vi "Encoder Test.vi"() -> ()   [LabVIEW 2011]
uses:
  <vilib>/Rock Robotics/SystemInterfaces/DIO/FPGA_DIOChannel.ctl
  <vilib>/Rock Robotics/SystemInterfaces/DIO/FPGA_DIOPWMChannel.ctl
  <vilib>/Rock Robotics/WPI/Joystick/WPI_JoystickDeviceEnum.ctl
  <vilib>/Rock Robotics/WPI/Encoder/WPI_EncoderType.ctl
  <vilib>/Rock Robotics/SystemInterfaces/Typedef/FPGA_TypedefDigitalModule.ctl
  <vilib>/Rock Robotics/SystemInterfaces/Typedef/FPGA_TypedefAnalogModule.ctl
  <vilib>/Rock Robotics/SystemInterfaces/AI/FPGA_AIChannel.ctl
  <vilib>/Rock Robotics/WPI/Counter/WPI_CounterDigitalInputToDigitalSource.vi
  <vilib>/Rock Robotics/WPI/MotorControl/WPI_MotorControlOpen Jaguar.vi
  <vilib>/Rock Robotics/WPI/Counter/WPI_CounterOpen UpDown Mode.vi
panel:
  out "period":dbl
  out "Numeric":dbl
  out "Average":dbl
  out "Voltage":dbl(knob) scale=30.0..80.0
  out "RPM 2":dbl(knob) scale=0.0..6000.0
  in  "Knob":dbl(knob) scale=0.0..1.0
  out "Gauge 2":dbl(knob) scale=-100.0..100.0
  in  "stop":bool
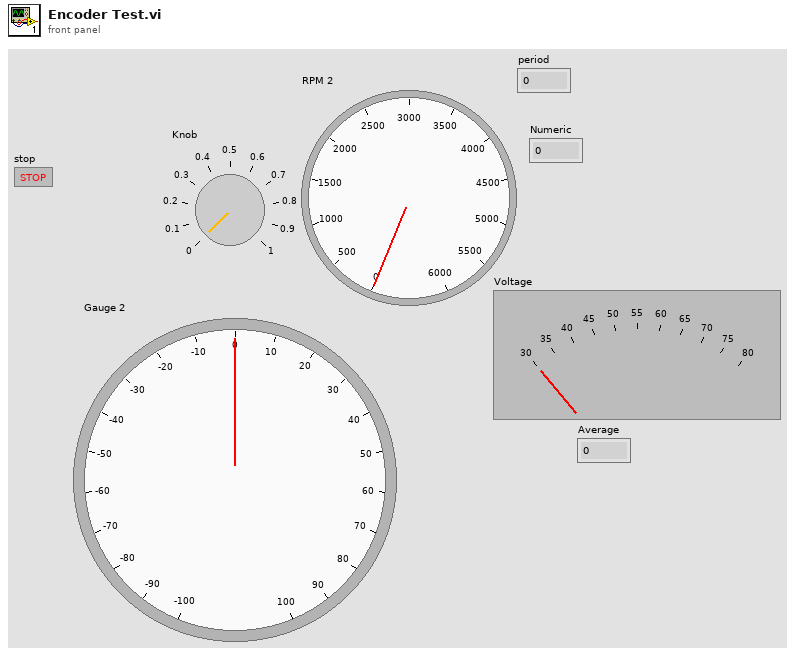
[diagram p1: front panel]
types:
  T1 = typedef "FPGA_AIChannel.ctl" = enum8{"AI 1", "AI 2", "AI 3", "AI 4", "AI 5", "AI 6", "AI 7", "AI 8", "Invalid"}
  T2 = typedef "FPGA_TypedefAnalogModule.ctl" = enum16{"Analog Module 1", "Analog Module 2"}
  T3 = typedef "FPGA_DIOChannel.ctl" = enum8{"DIO 1", "DIO 2", "DIO 3", "DIO 4", "DIO 5", "DIO 6", "DIO 7", "DIO 8", "DIO 9", "DIO 10", "DIO 11", "DIO 12", "DIO 13", "DIO 14", "Invalid"}
  T4 = typedef "FPGA_TypedefDigitalModule.ctl" = enum16{"Digital Module 1", "Digital Module 2"}
  T5 = typedef "WPI_EncoderType.ctl" = enum16{"1x", "2x", "4x"}
  T6 = typedef "FPGA_DIOPWMChannel.ctl" = enum8{"PWM 1", "PWM 2", "PWM 3", "PWM 4", "PWM 5", "PWM 6", "PWM 7", "PWM 8", "PWM 9", "PWM 10", "Invalid"}
  T7 = typedef "WPI_JoystickDeviceEnum.ctl" = enum16{"USB 1", "USB 2", "USB 3", "USB 4", "Kinect 1", "Kinect 2"}
  T8 = typedef "WPI_DigitalInputDevRef.ctl" = cluster{"DevStatus":errorcluster, "DIO Channel":T3, "Digital Module":T4}
  T9 = typedef "FPGA_CounterEncoderSourceConvertionLVSourceType.ctl" = cluster{"DevStatus":errorcluster, "AnalogTriggerMode?":bool, "DigitalMode":cluster{"Digital Module":T4, "DIO Channel":T10}, "AnalogTriggerMode":cluster{"AnalogTriggerIndex":T11, "OutputType":T12}}
  T10 = typedef "FPGA_DIODigitalSourceChannel.ctl" = enum8{"DIO 1", "DIO 2", "DIO 3", "DIO 4", "DIO 5", "DIO 6", "DIO 7", "DIO 8", "DIO 9", "DIO 10", "DIO 11", "DIO 12", "DIO 13", "DIO 14", "Disabled"}
  T11 = typedef "FPGA_AnalogTriggerIndex.ctl" = enum8{"Trig 0", "Trig 1", "Trig 2", "Trig 3", "Trig 4", "Trig 5", "Trig 6", "Trig 7", "Invalid"}
  T12 = typedef "FPGA_AnalogTriggerOutType.ctl" = enum16{"InWindow", "TriggerState", "Rising", "Falling"}
  T13 = typedef "WPI_EncoderDevRef.ctl" = cluster{"DevStatus":errorcluster, "EncoderIndex":T14, "CounterIndex":T15, "DistancePerCount":dbl, "Decoding Type":T5}
  T14 = typedef "FPGA_EncoderIdx.ctl" = enum8{"Enc 0", "Enc 1", "Enc 2", "Enc 3", "Invalid"}
  T15 = typedef "FPGA_CounterCtrSystemIndex.ctl" = enum8{"Ctr 0", "Ctr 1", "Ctr 2", "Ctr 3", "Ctr 4", "Ctr 5", "Ctr 6", "Ctr 7", "Invalid"}
  T16 = typedef "WPI_CounterDevRef.ctl" = cluster{"DevStatus":errorcluster, "CntIndex":T15}
  T17 = typedef "WPI_MotorControlDeviceRef.ctl" = cluster{"DeviceStatus":errorcluster, "Type":enum16{"PWM", "CAN"}, "PWM":cluster{"Digital Module":T4, "PWM Channel":T6, "DeadBand":T18}, "CAN":cluster{"Device Number":u8, "Control Mode":T19, "Semaphore":T20, "Max Vout":dbl}, "Invert":bool, "TransformRef":T21, "InvTransformRef":T21}
  T18 = typedef "WPI_PWMDeadband.ctl" = cluster{"Name":string, "maxPositivePwm":i32, "minPositivePwm":i32, "centerPwm":i32, "maxNegativePwm":i32, "minNegativePwm":i32, "angularRange":u16}
  T19 = typedef "WPI_CANJaguar_ControlMode.ctl" = enum8{"Percent VBus", "Current", "Speed", "Position", "Voltage"}
  T20 = typedef "Semaphore RefNum" = refnum<k1>
  T21 = typedef "WPI_PWMTransform_ConPane.ctl" = refnum<vi>
  T22 = typedef "WPI_AnalogChannelDevRef.ctl" = cluster{"DevStatus":errorcluster, "Analog Module":T2, "Analog Channel":T1}
  T23 = typedef "WPI_JoystickDevRef.ctl" = cluster{"Device":T7}
  T24 = typedef "WPI_JoystickButtonState.ctl" = cluster{"Button 1":bool, "Button 2":bool, "Button 3":bool, "Button 4":bool, "Button 5":bool, "Button 6":bool, "Button 7":bool, "Button 8":bool, "Button 9":bool, "Button 10":bool, "Button 11":bool, "Button 12":bool}
  T25 = cluster{"axis 1 (x)":dbl, "axis 2 (y)":dbl, "axis 3 (throttle)":dbl, "axis 4":dbl, "axis 5":dbl, "axis 6":dbl}
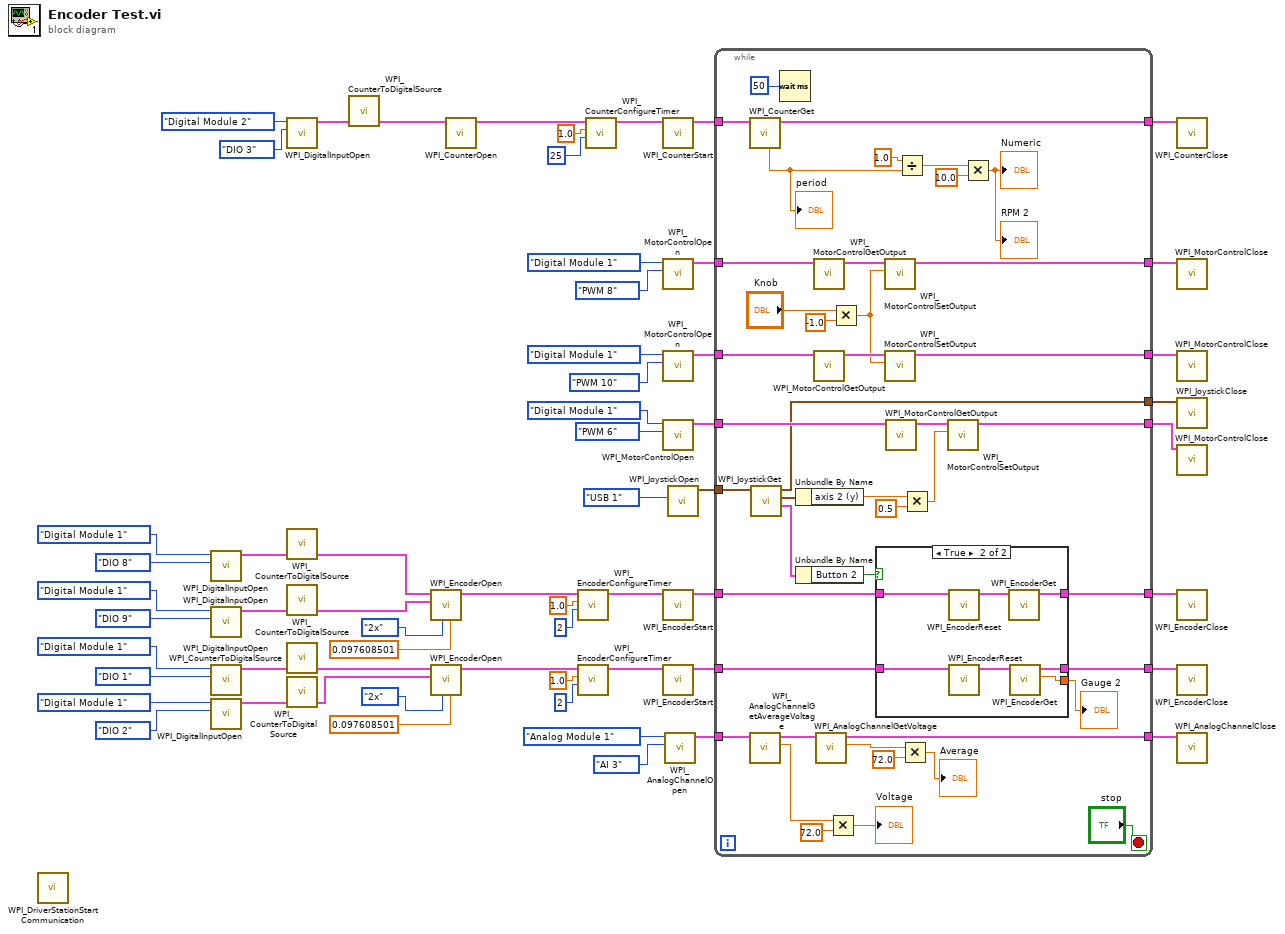
[diagram p0: block diagram]
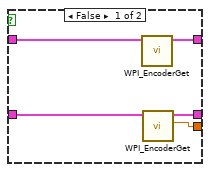
[diagram p2: hidden frame]
diagram:
  n1 = call <vilib>:"WPI_DriverStationStart Communication.vi"() -> ()  [unwired: 12 in]
  n2 = call <vilib>:"WPI_DigitalInputOpen.vi"("DIO Channel"=FPGA_DIOChannel."DIO 8", "Digital Module (Module 1)"=FPGA_TypedefDigitalModule."Digital Module 1") -> ("DigitalInputDevRef"=w58:T8)  [unwired: 8 in, 1 out]
  n3 = call <vilib>:"WPI_DigitalInputOpen.vi"("DIO Channel"=FPGA_DIOChannel."DIO 9", "Digital Module (Module 1)"=FPGA_TypedefDigitalModule."Digital Module 1") -> ("DigitalInputDevRef"=w61:T8)  [unwired: 8 in, 1 out]
  n4 = call <vilib>:"WPI_DigitalInputOpen.vi"("DIO Channel"=FPGA_DIOChannel."DIO 1", "Digital Module (Module 1)"=FPGA_TypedefDigitalModule."Digital Module 1") -> ("DigitalInputDevRef"=w22:T8)  [unwired: 8 in, 1 out]
  n5 = call <vilib>:"WPI_DigitalInputOpen.vi"("DIO Channel"=FPGA_DIOChannel."DIO 2", "Digital Module (Module 1)"=FPGA_TypedefDigitalModule."Digital Module 1") -> ("DigitalInputDevRef"=w19:T8)  [unwired: 8 in, 1 out]
  n6 = call <vilib>:"WPI_DigitalInputOpen.vi"("DIO Channel"=FPGA_DIOChannel."DIO 3", "Digital Module (Module 1)"=FPGA_TypedefDigitalModule."Digital Module 2") -> ("DigitalInputDevRef"=w11:T8)  [unwired: 8 in, 1 out]
  n7 = call-poly <vilib>:"WPI_CounterToDigitalSource.vi"("DigitalInputDevRef"=w58) -> ("Digital Source"=w59:T9)  [unwired: 6 in]
  n8 = call-poly <vilib>:"WPI_CounterToDigitalSource.vi"("DigitalInputDevRef"=w61) -> ("Digital Source"=w60:T9)  [unwired: 6 in]
  n9 = call-poly <vilib>:"WPI_CounterToDigitalSource.vi"("DigitalInputDevRef"=w22) -> ("Digital Source"=w21:T9)  [unwired: 6 in]
  n10 = call-poly <vilib>:"WPI_CounterToDigitalSource.vi"("DigitalInputDevRef"=w19) -> ("Digital Source"=w20:T9)  [unwired: 6 in]
  n11 = call-poly <vilib>:"WPI_CounterToDigitalSource.vi"("DigitalInputDevRef"=w11) -> ("Digital Source"=w12:T9)  [unwired: 6 in]
  n12 = call <vilib>:"WPI_EncoderOpen.vi"("DistancePerCount"=0.097608501, "Decoding Type"=WPI_EncoderType."2x", "BSource"=w60, "ASource"=w59) -> ("EncoderDevRef"=w53:T13)  [unwired: 6 in, 1 out]
  n13 = call <vilib>:"WPI_EncoderOpen.vi"("DistancePerCount"=0.097608501, "Decoding Type"=WPI_EncoderType."2x", "BSource"=w20, "ASource"=w21) -> ("EncoderDevRef"=w27:T13)  [unwired: 6 in, 1 out]
  n14 = call-poly <vilib>:"WPI_CounterOpen.vi"("Up Source"=w12) -> ("CounterDevRef"=w16:T16)  [unwired: 9 in, 1 out]
  n15 = call <vilib>:"WPI_EncoderConfigureTimer.vi"("Number Samples to Average"=u8 2, "Minimum Rate"=1.0, "EncoderDevRef"=w53) -> ("EncoderDevRef"=w52:T13)  [unwired: 7 in, 1 out]
  n16 = call <vilib>:"WPI_EncoderConfigureTimer.vi"("Number Samples to Average"=u8 2, "Minimum Rate"=1.0, "EncoderDevRef"=w27) -> ("EncoderDevRef"=w28:T13)  [unwired: 7 in, 1 out]
  n17 = call <vilib>:"WPI_CounterConfigureTimer.vi"("Number Samples to Average"=u8 25, "MaxPeriod (sec)"=1.0, "CounterDevRef in"=w16) -> ("CounterDevRef out"=w15:T16)  [unwired: 7 in, 1 out]
  n18 = call <vilib>:"WPI_CounterStart.vi"("CounterDevRef in"=w15) -> ("CounterDevRef out"=w14:T16)  [unwired: 9 in, 1 out]
  n19 = call-poly <vilib>:"WPI_MotorControlOpen.vi"("PWM Channel"=FPGA_DIOPWMChannel."PWM 8", "Digital Module (Module 1)"=FPGA_TypedefDigitalModule."Digital Module 1") -> ("MotorControlDeviceRef"=w36:T17)  [unwired: 8 in, 1 out]
  n20 = call-poly <vilib>:"WPI_MotorControlOpen.vi"("PWM Channel"=FPGA_DIOPWMChannel."PWM 10", "Digital Module (Module 1)"=FPGA_TypedefDigitalModule."Digital Module 1") -> ("MotorControlDeviceRef"=w33:T17)  [unwired: 8 in, 1 out]
  n21 = call-poly <vilib>:"WPI_MotorControlOpen.vi"("PWM Channel"=FPGA_DIOPWMChannel."PWM 6", "Digital Module (Module 1)"=FPGA_TypedefDigitalModule."Digital Module 1") -> ("MotorControlDeviceRef"=w43:T17)  [unwired: 8 in, 1 out]
  n22 = call <vilib>:"WPI_EncoderStart.vi"("EncoderDevRef"=w52) -> ("EncoderDevRef"=w51:T13)  [unwired: 9 in, 1 out]
  n23 = call <vilib>:"WPI_EncoderStart.vi"("EncoderDevRef"=w28) -> ("EncoderDevRef"=w18:T13)  [unwired: 9 in, 1 out]
  n24 = call <vilib>:"WPI_AnalogChannelOpen.vi"("Analog Channel"=FPGA_AIChannel."AI 3", "Analog Module (Module 1)"=FPGA_TypedefAnalogModule."Analog Module 1") -> ("AIDeviceRef"=w6:T22)  [unwired: 8 in, 1 out]
  n25 = call <vilib>:"WPI_JoystickOpen.vi"("JoystickDevice"=WPI_JoystickDeviceEnum."USB 1") -> ("JoystickDevRef"=w40:T23)  [unwired: 10 in]
  n26 = while {
    tunnel: w51 -> [w95]
    tunnel: [w104] -> w50
    tunnel: w43 -> [w101]
    tunnel: [w100] -> w42
    tunnel: [w99] -> w41
    tunnel: w40 -> [w97]
    tunnel: w36 -> [w92]
    tunnel: w33 -> [w90]
    tunnel: w18 -> [w89]
    tunnel: [w88] -> w17
    tunnel: w14 -> [w86]
    tunnel: [w85] -> w13
    tunnel: w6 -> [w80]
    tunnel: [w78] -> w5
    tunnel: [w64] -> w2
    tunnel: [w63] -> w1
    stop <- "stop" stop-if-true
    n27 = call <vilib>:"WPI_CounterGet.vi"("CounterDevRef in"=w86) -> ("CounterDevRef out"=w85:T16, "Period (sec)"=w62:dbl)  [unwired: 5 in, 4 out]
    "period" <- w62
    n28 = call <vilib>:"WPI_AnalogChannelGetAverageVoltage.vi"("AIDeviceRef"=w80) -> ("Voltage"=w76:dbl, "AIDeviceRef"=w79:T22)  [unwired: 8 in, 1 out]
    n29 = call <vilib>:"WPI_JoystickGet.vi"("JoystickDevRef"=w97) -> ("Buttons"=w96:T24, "Axes"=w98:T25, "JoystickDevRef"=w99:T23)  [unwired: 4 in]
    n30 = Wait (ms)(milliseconds to wait=u32 50) -> ()  [unwired: 1 out]
    n31 = Unbundle By Name(w98) -> ("axis 2 (y)"=w69:dbl)
    n32 = Unbundle By Name(w96) -> ("Button 2"=w94:bool)
    n33 = call <vilib>:"WPI_MotorControlGetOutput.vi"("MotorControlDevRef"=w92) -> ("MotorControlDevRef"=w93:T17)  [unwired: 8 in, 2 out]
    n34 = call <vilib>:"WPI_MotorControlGetOutput.vi"("MotorControlDevRef"=w90) -> ("MotorControlDevRef"=w91:T17)  [unwired: 8 in, 2 out]
    n35 = call <vilib>:"WPI_AnalogChannelGetVoltage.vi"("AIDeviceRef"=w79) -> ("Voltage"=w73:dbl, "AIDeviceRef"=w78:T22)  [unwired: 8 in, 1 out]
    n36 = Multiply(x=w76, y=72.0) -> (x*y=→"Voltage":dbl)
    n37 = Multiply(x="Knob", y=-1.0) -> (x*y=w65:dbl)
    n38 = case shown="True" w94 {
      tunnel: [w108 w116] -> w104
      tunnel: w95 -> [w109 w115]
      tunnel: w89 -> [w106 w112]
      tunnel: [w107 w111] -> w88
      tunnel: [w105 w110] -> w87
      frame False {
        n39 = call <vilib>:"WPI_EncoderGet.vi"("EncoderDevRef"=w109) -> ("EncoderDevRef"=w108:T13)  [unwired: 5 in, 5 out]
        n40 = call <vilib>:"WPI_EncoderGet.vi"("EncoderDevRef"=w106) -> ("Distance"=w105:dbl, "EncoderDevRef"=w107:T13)  [unwired: 5 in, 4 out]
      }
      frame True {
        n41 = call <vilib>:"WPI_EncoderReset.vi"("EncoderDevRef"=w115) -> ("EncoderDevRef"=w114:T13)  [unwired: 9 in, 1 out]
        n42 = call <vilib>:"WPI_EncoderReset.vi"("EncoderDevRef"=w112) -> ("EncoderDevRef"=w113:T13)  [unwired: 9 in, 1 out]
        n43 = call <vilib>:"WPI_EncoderGet.vi"("EncoderDevRef"=w114) -> ("EncoderDevRef"=w116:T13)  [unwired: 5 in, 5 out]
        n44 = call <vilib>:"WPI_EncoderGet.vi"("EncoderDevRef"=w113) -> ("Distance"=w110:dbl, "EncoderDevRef"=w111:T13)  [unwired: 5 in, 4 out]
      }
    }
    "Gauge 2" <- w87
    n45 = call <vilib>:"WPI_MotorControlSetOutput.vi"("Output"=w65, "MotorControlDevRef"=w93) -> ("MotorControlDevRef"=w64:T17)  [unwired: 8 in, 1 out]
    n46 = call <vilib>:"WPI_MotorControlSetOutput.vi"("Output"=w65, "MotorControlDevRef"=w91) -> ("MotorControlDevRef"=w63:T17)  [unwired: 8 in, 1 out]
    n47 = call <vilib>:"WPI_MotorControlGetOutput.vi"("MotorControlDevRef"=w101) -> ("MotorControlDevRef"=w102:T17)  [unwired: 8 in, 2 out]
    n48 = Divide(x=1.0, y=w62) -> (x/y=w83:dbl)
    n49 = Multiply(x=w73, y=72.0) -> (x*y=→"Average":dbl)
    n50 = Multiply(x=w69, y=0.5) -> (x*y=w68:dbl)
    n51 = call <vilib>:"WPI_MotorControlSetOutput.vi"("Output"=w68, "MotorControlDevRef"=w102) -> ("MotorControlDevRef"=w100:T17)  [unwired: 8 in, 1 out]
    n52 = Multiply(x=w83, y=10.0) -> (x*y=→"RPM 2" →"Numeric":dbl)
  }
  n53 = call <vilib>:"WPI_CounterClose.vi"("CounterDevRef"=w13) -> ()  [unwired: 10 in, 1 out]
  n54 = call <vilib>:"WPI_MotorControlClose.vi"("MotorControlDevRef"=w2) -> ()  [unwired: 10 in, 1 out]
  n55 = call <vilib>:"WPI_MotorControlClose.vi"("MotorControlDevRef"=w1) -> ()  [unwired: 10 in, 1 out]
  n56 = call <vilib>:"WPI_JoystickClose.vi"("JoystickDevRef"=w41) -> ()  [unwired: 11 in]
  n57 = call <vilib>:"WPI_MotorControlClose.vi"("MotorControlDevRef"=w42) -> ()  [unwired: 10 in, 1 out]
  n58 = call <vilib>:"WPI_EncoderClose.vi"("EncoderDevRef"=w50) -> ()  [unwired: 10 in, 1 out]
  n59 = call <vilib>:"WPI_EncoderClose.vi"("EncoderDevRef"=w17) -> ()  [unwired: 10 in, 1 out]
  n60 = call <vilib>:"WPI_AnalogChannelClose.vi"("AIDeviceRef"=w5) -> ()  [unwired: 10 in, 1 out]
